vi "Write_to_server.vi"() -> ()   [LabVIEW 2023]
panel:
  in  "Time interval":u32=100
  out "OPC URLs":string[](array[string])
  in  "Number of tags to read from":i32
  in  "Data to write to server":dbl[](array[numeric])
  in  "Stop Button":bool
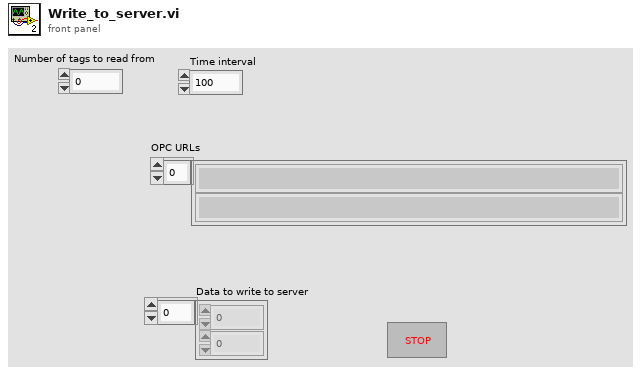
[diagram p1: front panel]
types:
  T1 = enum16{"Read", "Write", "ReadWrite", "BufferedRead", "BufferedReadWrite"}
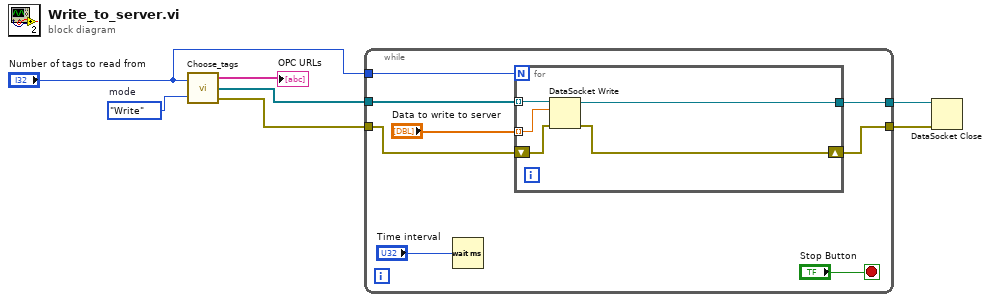
[diagram p0: block diagram]
diagram:
  w5 = T1."Write"  # mode
  n1 = call "Choose_tags.vi"("Number of tags to read from"="Number of tags to read from", "mode"=w5) -> ("Tags opened"=→"OPC URLs":string[], "Opened tags refnumbers"=w3:refnum<k13>[], "error out"=w2:errorcluster)
  n2 = while {
    tunnel: w3 -> [w15]
    tunnel: w2 -> [w13]
    tunnel: [w12] -> w7
    tunnel: [w11] -> w6
    tunnel: "Number of tags to read from" -> [w8]
    stop <- "Stop Button" stop-if-true
    n3 = Wait (ms)(milliseconds to wait="Time interval") -> ()  [unwired: 1 out]
    n4 = for {
      N: w8 -> [_]
      tunnel: w15 -> [w20] mode=indexing
      tunnel: [w17] -> w11
      tunnel: "Data to write to server" -> [w16] mode=indexing
      shift-right: [w18] -> w12
      shift-left: w13 -> [w19]
      n5 = DataSocket Write(8:w19, 10:w16, 11:w20) -> (0:w18:errorcluster, 3:w17:refnum<k13>)  [unwired: 1 in, 1 out]
    }
  }
  n6 = DataSocket Close(8:w7, 11:w6) -> ()  [unwired: 1 in, 2 out]
